vi "Database.Main.Disconnect.vi"(8 "error in (no error)":errorcluster, 11 "Data in":T1 {"Variant"."TS"."TV"."minimum" format="%#.3f"; "Variant"."TS"."TV"."maximum" format="%#.3f"; "Variant"."TS"."TP"."value" format="%#.3f"}) -> (0 "error out":errorcluster, 3 "Data out":T1 {"Variant"."TS"."TV"."minimum" format="%#.3f"; "Variant"."TS"."TV"."maximum" format="%#.3f"; "Variant"."TS"."TP"."value" format="%#.3f"})   [LabVIEW 2016]
doc: "Disconnect from database\n\nWabco 2017 All right reserved\nAuthor: maciej.szupienko@wabco-auto.com"
uses:
  Database.Main.Data.ctl
  Database.Main.Data.Status.ctl
  Database.Main.Data.Sets.ctl
  Database.Main.Data.Results.ctl
  ProdaNG/Controls/ProdaNG.Identification.ctl
  ProdaNG/Controls/ProdaNG.ProcessResult.ctl
  ProdaNG/Controls/ProdaNG.ProcessStepResult.ctl
  ProdaNG/Controls/ProdaNG.TestStepResult.ctl
  ProdaNG/Controls/ProdaNG.TestValueResult.ctl
  Database.Main.Data.Variant.ctl
  ProdaNG/Controls/ProdaNG.ProcessStepParam.ctl
  ProdaNG/Controls/ProdaNG.TestStep.ctl
  ProdaNG/Controls/ProdaNG.TestStepParam.ctl
  ProdaNG/Controls/ProdaNG.TestValue.ctl
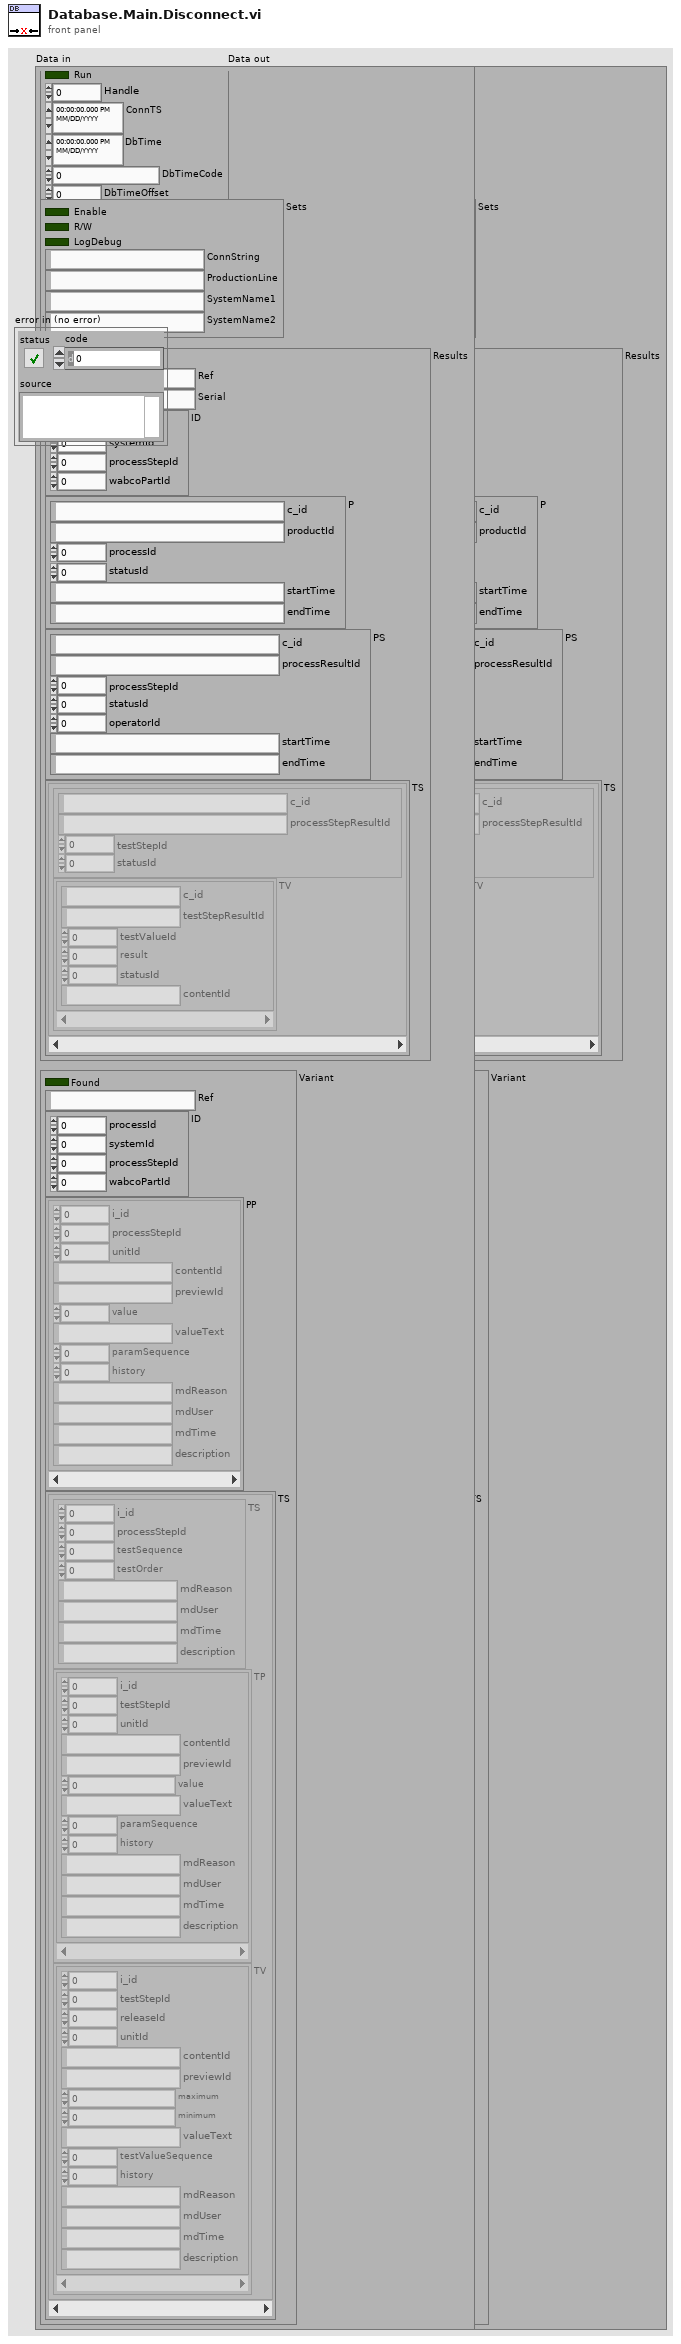
[diagram p1: front panel]
types:
  T1 = typedef "Database.Main.Data.ctl" = cluster{"Status":T2, "Sets":T3, "Results":T4, "Variant":T10}
  T2 = typedef "Database.Main.Data.Status.ctl" = cluster{"Run":bool, "Handle":i32, "ConnTS":timestamp, "DbTime":timestamp, "DbTimeCode":dbl, "DbTimeOffset":dbl}
  T3 = typedef "Database.Main.Data.Sets.ctl" = cluster{"Enable":bool, "R/W":bool, "LogDebug":bool, "ConnString":string, "ProductionLine":string, "SystemName1":string, "SystemName2":string}
  T4 = typedef "Database.Main.Data.Results.ctl" = cluster{"Service":bool, "Ref":string, "Serial":string, "ID":T5, "P":T6, "PS":T7, "TS":cluster{"TS":T8, "TV":T9[]}[]}
  T5 = typedef "ProdaNG.Identification.ctl" = cluster{"processId":i32, "systemId":i32, "processStepId":i32, "wabcoPartId":i32}
  T6 = typedef "ProdaNG.ProcessResult.ctl" = cluster{"c_id":string, "productId":string, "processId":i32, "statusId":i32, "startTime":string, "endTime":string}
  T7 = typedef "ProdaNG.ProcessStepResult.ctl" = cluster{"c_id":string, "processResultId":string, "processStepId":i32, "statusId":i32, "operatorId":i32, "startTime":string, "endTime":string}
  T8 = typedef "ProdaNG.TestStepResult.ctl" = cluster{"c_id":string, "processStepResultId":string, "testStepId":i32, "statusId":i32}
  T9 = typedef "ProdaNG.TestValueResult.ctl" = cluster{"c_id":string, "testStepResultId":string, "testValueId":i32, "result":dbl, "statusId":i32, "contentId":string}
  T10 = typedef "Database.Main.Data.Variant.ctl" = cluster{"Found":bool, "Ref":string, "ID":T5, "PP":T11[], "TS":cluster{"TS":T12, "TP":T13[], "TV":T14[]}[]}
  T11 = typedef "ProdaNG.ProcessStepParam.ctl" = cluster{"i_id":i32, "processStepId":i32, "unitId":i32, "contentId":string, "previewId":string, "value":dbl, "valueText":string, "paramSequence":i32, "history":i32, "mdReason":string, "mdUser":string, "mdTime":string, "description":string}
  T12 = typedef "ProdaNG.TestStep.ctl" = cluster{"i_id":i32, "processStepId":i32, "testSequence":i32, "testOrder":i32, "mdReason":string, "mdUser":string, "mdTime":string, "description":string}
  T13 = typedef "ProdaNG.TestStepParam.ctl" = cluster{"i_id":i32, "testStepId":i32, "unitId":i32, "contentId":string, "previewId":string, "value":dbl, "valueText":string, "paramSequence":i32, "history":i32, "mdReason":string, "mdUser":string, "mdTime":string, "description":string}
  T14 = typedef "ProdaNG.TestValue.ctl" = cluster{"i_id":i32, "testStepId":i32, "releaseId":i32, "unitId":i32, "contentId":string, "previewId":string, "maximum":dbl, "minimum":dbl, "valueText":string, "testValueSequence":i32, "history":i32, "mdReason":string, "mdUser":string, "mdTime":string, "description":string}
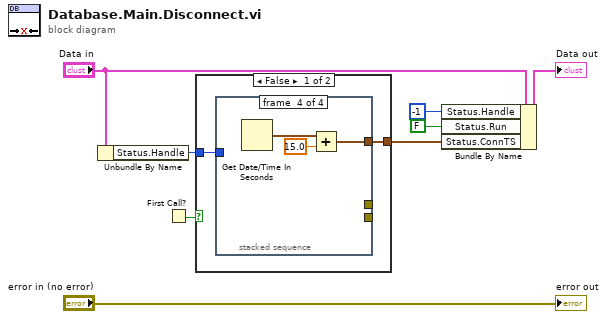
[diagram p0: block diagram]
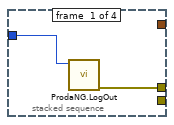
[diagram p2: hidden frame]
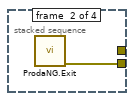
[diagram p3: hidden frame]
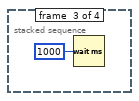
[diagram p4: hidden frame]
diagram:
  n1 = Unbundle By Name("Data in") -> ("Status.Handle"=w6:i32)
  n2 = First Call?() -> (First Call?: T/F=w1:bool)
  n3 = case shown="False" w1 {
    tunnel: w6 -> [w10 _]
    tunnel: [w9 _] -> w3
    frame False {
      n4 = stacked-sequence {
        tunnel: w10 -> [w12 _ _ _]
        tunnel: [w11 _ _ _] -> _
        tunnel: [_ _ _ w15] -> w9
        tunnel: [_ w13 _ _] -> _
        frame #0 {
          n5 = call "ProdaNG.LogOut.vi"("dbHandleIn"=w12) -> ("error out"=w11:errorcluster)  [unwired: 10 in]
        }
        frame #1 {
          n6 = call "ProdaNG.Exit.vi"() -> ("error out"=w13:errorcluster)  [unwired: 11 in]
        }
        frame #2 {
          n7 = Wait (ms)(milliseconds to wait=u32 1000) -> ()  [unwired: 1 out]
        }
        frame #3 {
          n8 = Get Date/Time In Seconds() -> (seconds since 1Jan1904=w17:timestamp)
          n9 = Add(x=w17, y=15.0) -> (x+y=w15:timestamp)
        }
      }
    }
    frame True {
    }
  }
  n10 = Bundle By Name(cluster="Data in", "Status.Handle"=-1, "Status.Run"=FALSE ("Status.Connected"), "Status.ConnTS"=w3) -> (→"Data out":T1)
  "error out" <- "error in (no error)"
